vi "NI_SAT_TEST_20150519_EXP_V3_SINWAVE.vi"() -> ()   [LabVIEW 2013]
uses:
  <instrlib>/niFgen/niFgen.llb/niFgen Waveform Type.ctl
  <instrlib>/niFgen/niFgen.llb/niFgen Output Impedance.ctl
  <vilib>/Waveform/WDTOps.llb/WDT Append Waveforms DBL.vi
panel:
  out "appended array":dbl[](array[numeric])
  in  "amplitude":dbl=1.0 format="%#_3p"
  in  "frequency":dbl=1000000.0 format="%#_12p"
  in  "waveform":T1=5 caption="Waveform" items=["Sine", "Square", "Triangle", "Ramp Up", "Ramp Down", "DC", "Noise", "User"]
  out "Tabs 1 Through # Used":i32
  in  "Tab Control 3":T2(tab)
  out "Tab Control 2":T2(tab)
  out "Waveform Graph 1":waveform(dbl)(graph)
  out "Waveform Graph 2":waveform(dbl)(graph)
  out "Waveform Graph 3":waveform(dbl)(graph)
  out "Waveform Graph 4":waveform(dbl)(graph)
  out "Waveform Graph 5":waveform(dbl)(graph)
  out "Waveform Graph 6":waveform(dbl)(graph)
  out "Waveform Graph 7":waveform(dbl)(graph)
  out "Waveform Graph 8":waveform(dbl)(graph)
  out "Waveform Graph 9":waveform(dbl)(graph)
  out "Waveform Graph 10":waveform(dbl)(graph)
  out "Waveform Graph 11":waveform(dbl)(graph)
  out "Waveform Graph 12":waveform(dbl)(graph)
  out "Waveform Graph 13":waveform(dbl)(graph)
  out "Waveform Graph 14":waveform(dbl)(graph)
  out "Waveform Graph 15":waveform(dbl)(graph)
  out "Waveform Graph 16":waveform(dbl)(graph)
  out "Waveform Graph 17":waveform(dbl)(graph)
  out "Waveform Graph 18":waveform(dbl)(graph)
  out "Waveform Graph 19":waveform(dbl)(graph)
  out "Waveform Graph 20":waveform(dbl)(graph)
  out "Diff in Methods before call DMM vi and before read Wave Data (SEC)":dbl
  out "Total Elapsed Time (ms)":u32
  out "TotalElapsed Time (Sec)":dbl
  out "Waveform Graph":waveform(dbl)(graph)
  in  "Output Voltage Division":i32
  in  "Highest Output Voltage [Volts]":i32 min=-600 max=600 step=20
  in  "Rate":dbl=10.0 caption="Rate (Samples/Sec)" format="%.2f"
  in  "Waveform Points":i32=101 caption="Samples"
  in  "Function Generator Name":refnum<k15>="PXI1Slot2"
  # "Please Enter Output Voltage\nwith the desired sign. Be it positive\nor negative. Program will divide 200 and then negate, due to gain of 200 and inversion of input by amplifier"
  # "ENJOY PETER, still could use tweeking to make it run smoother and prevent more user error, but meh. Goodmorning"
  # "Output voltage comes from the VOLTAGE MONITOR (VM) from the amplifier with (1V VM/200V AMP)"
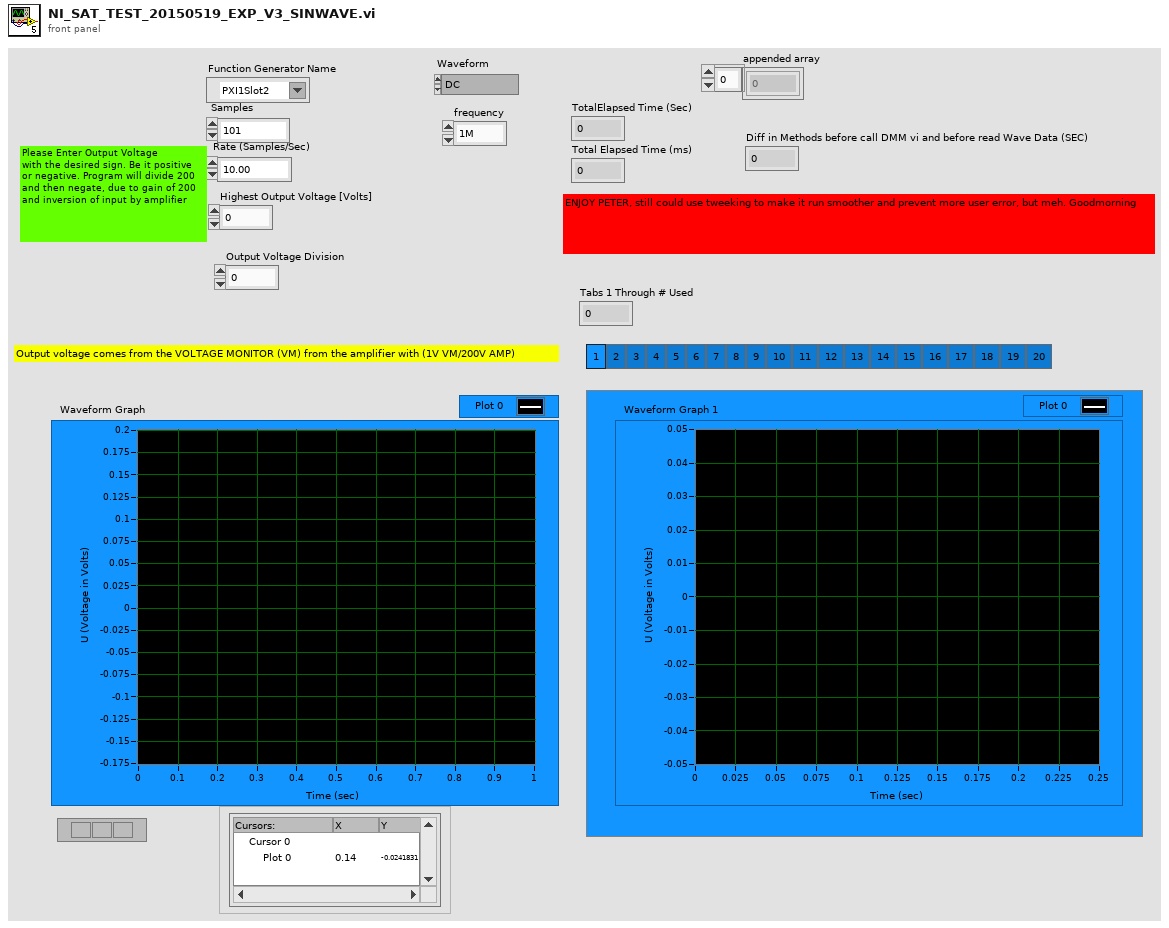
[diagram p1: front panel]
types:
  T1 = typedef "niFgen Waveform Type.ctl" = i32
  T2 = enum32{"1", "2", "3", "4", "5", "6", "7", "8", "9", "10", "11", "12", "13", "14", "15", "16", "17", "18", "19", "20"}
  T3 = enum16{"open", "replace", "create", "open or create", "replace or create", "replace or create with confirmation"}
  T4 = typedef "niFgen Output Impedance.ctl" = i32
  T5 = cluster{"channel name":string, "waveform":T1, "frequency":dbl, "y":dbl, "start phase":dbl, "dc offset":dbl, "duty cycle high":i32, "impedance":T4, "load impedance":dbl}
  T6 = cluster{"channel name":string, "waveform":T1, "frequency":dbl, "y":dbl, "start phase":dbl, "dc offset":dbl, "duty cycle high":i32, "impedance":T4, "load impedance":dbl}[]
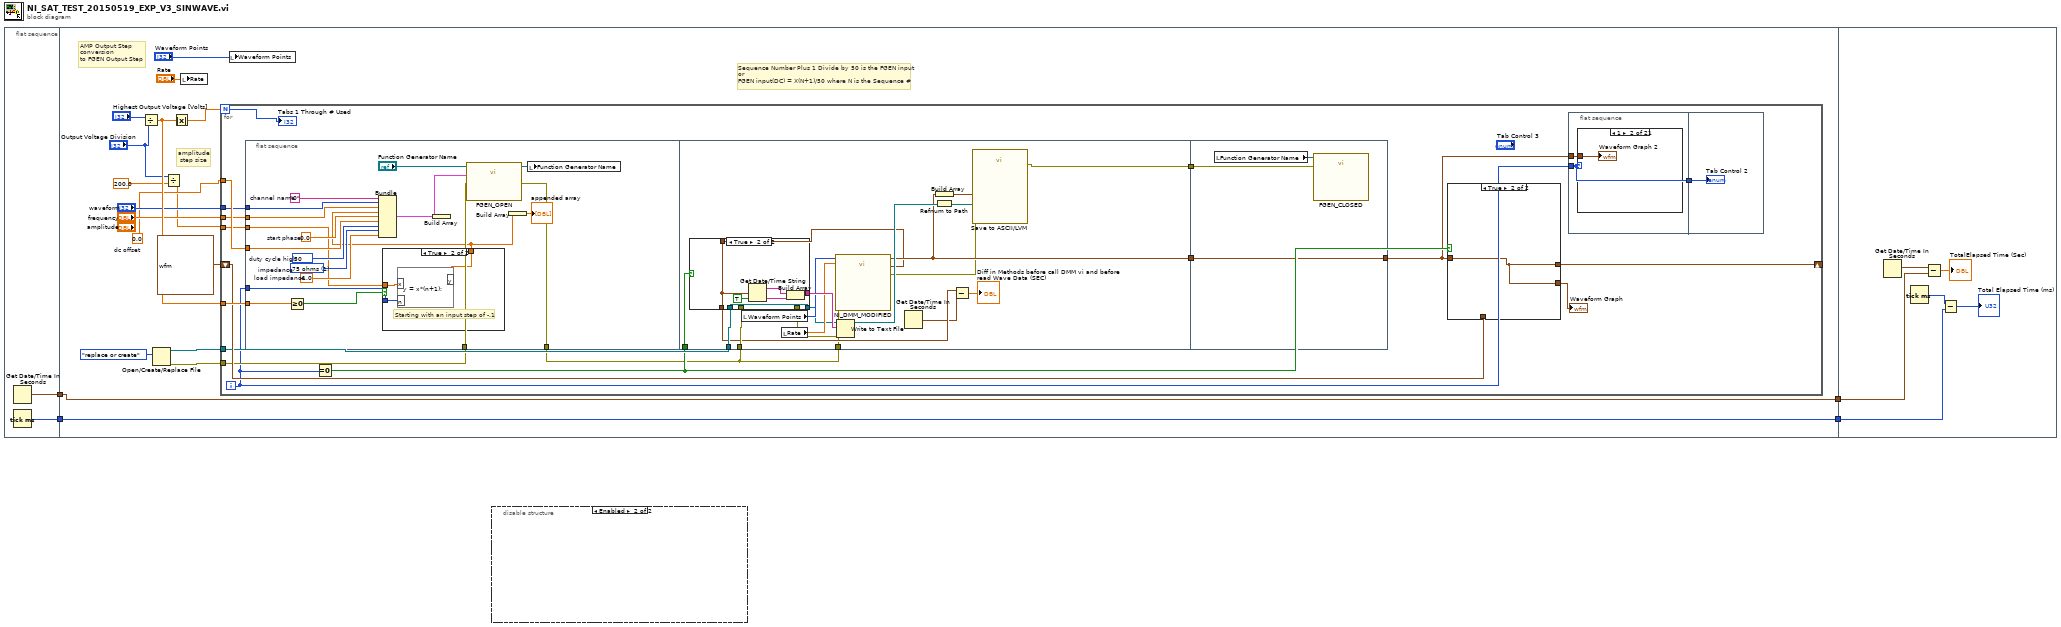
[diagram p0: block diagram]
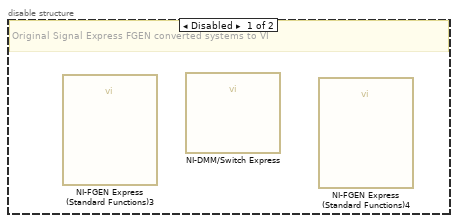
[diagram p2: hidden frame]
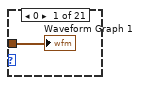
[diagram p3: hidden frame]
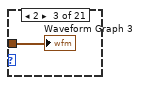
[diagram p4: hidden frame]
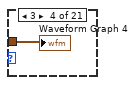
[diagram p5: hidden frame]
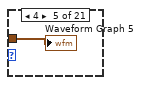
[diagram p6: hidden frame]
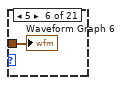
[diagram p7: hidden frame]
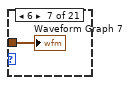
[diagram p8: hidden frame]
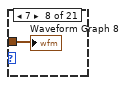
[diagram p9: hidden frame]
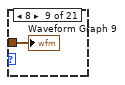
[diagram p10: hidden frame]
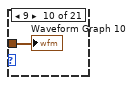
[diagram p11: hidden frame]
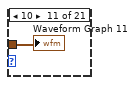
[diagram p12: hidden frame]
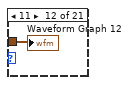
[diagram p13: hidden frame]
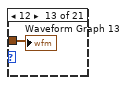
[diagram p14: hidden frame]
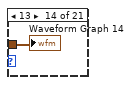
[diagram p15: hidden frame]
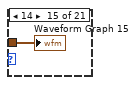
[diagram p16: hidden frame]
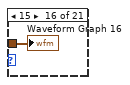
[diagram p17: hidden frame]
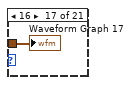
[diagram p18: hidden frame]
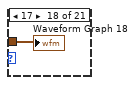
[diagram p19: hidden frame]
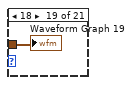
[diagram p20: hidden frame]
diagram:
  n1 = flat-sequence {
    tunnel: [w6] -> w4
    tunnel: [w5] -> w3
    tunnel: w4 -> [w15]
    tunnel: w3 -> [w14]
    tunnel: [w15] -> w2
    tunnel: [w14] -> w1
    tunnel: w2 -> [w136]
    tunnel: w1 -> [w135]
    frame #0 {
      n2 = Get Date/Time In Seconds() -> (seconds since 1Jan1904=w6:timestamp)
      n3 = Tick Count (ms)() -> (millisecond timer value=w5:u32)
    }
    frame #1 {
      w9 = 0.0  # dc offset
      # "AMP Output Step\nconversion\nto FGEN Output Step"
      # "amplitude\n step size"
      # "Sequence Number Plus 1 Divide by 50 is the FGEN input\nor\nFGEN input(DC) = X(N+1)/50 where N is the Sequence #"
      n4 = Divide(x="Highest Output Voltage [Volts]", y="Output Voltage Division") -> (x/y=w13:dbl)
      n5 = Open/Create/Replace File(operation (0:open)=T3."replace or create") -> (refnum out=w23:refnum<file>, error out=w22:errorcluster)  [unwired: 5 in, 1 out]
      n6 = Divide(x="Output Voltage Division", y=200.0) -> (x/y=w8:dbl)
      n7 = Absolute Value(x=w13) -> (abs(x)=w17:dbl)
      n8 = local write "Rate"("Rate") -> ()
      n9 = for {
        N: w17 -> [w29]
        tunnel: w23 -> [w37]
        tunnel: w22 -> [w34]
        tunnel: w13 -> [w40]
        shift-right: [w32] -> _
        shift-left: waveform(dbl) {"t0"=timestamp(0 s since 1904-01-01), "dt"=1.0, "Y"=[]} ("Waveform Data") -> [w39]
        tunnel: w9 -> [w27]
        tunnel: "waveform" -> [w26]
        tunnel: "frequency" -> [w25]
        tunnel: w8 -> [w24]
        i -> [w30]
        n10 = flat-sequence {
          tunnel: w30 -> [w82]
          tunnel: w40 -> [w79]
          tunnel: w34 -> [w77]
          tunnel: [w76] -> w33
          tunnel: w27 -> [w73]
          tunnel: w26 -> [w75]
          tunnel: w25 -> [w74]
          tunnel: w24 -> [w72]
          tunnel: [w109] -> w41
          tunnel: w36 -> [w106]
          tunnel: w37 -> [w105]
          tunnel: w33 -> [w103]
          tunnel: [w100] -> w35
          tunnel: w33 -> [w96]
          tunnel: w41 -> [w133]
          tunnel: [w133] -> w31
          tunnel: w35 -> [w132]
          frame #0 {
            w83 = -1.0  # load impedance
            w84 = T4 1 items=["50 ohms", "75 ohms", "1 mega ohm"]  # impedance
            w85 = 50  # duty cycle high
            w86 = 0.0  # start phase
            w71 = "0"  # channel name
            n11 = Greater Or Equal To 0?(x=w79) -> (x >= 0?=w78:bool)
            n12 = case shown="True" w78 {
              tunnel: w82 -> [w91 w94]
              tunnel: [w90 w93] -> w70
              tunnel: w72 -> [w89 w92]
              frame False {
                # "Starting with an input step of .1"
                # "Negative Output"
                n13 = formula code="y = -x*(n+1);"("x"=w89, "n"=w91) -> ("y"=w90:dbl)
              }
              frame True {
                # "Starting with an input step of -.1"
                n14 = formula code="y = x*(n+1);"("x"=w92, "n"=w94) -> ("y"=w93:dbl)
              }
            }
            n15 = Bundle("channel name"=w71, "waveform"=w75, "frequency"=w74, "y"=w70, "start phase"=w86, "dc offset"=w73, "duty cycle high"=w85, "impedance"=w84, "load impedance"=w83) -> (w81:T5)  [unwired: 1 in]
            n16 = Build Array(w81) -> (w80:T6)
            n17 = call "FGEN_OPEN.vi"("error in"=w77, "channel parameters"=w80, "resource name"="Function Generator Name") -> ("error out"=w76:errorcluster, "Instrument Handle Out"=w88:refnum<k15>)  [unwired: 7 in]
            n18 = Build Array(w70) -> (→"appended array":dbl[])
            n19 = local write "Function Generator Name"(w88) -> ()
          }
          frame #1 {
            n20 = local read "Waveform Points"() -> (w108:i32)
            n21 = local read "Rate"() -> (w107:dbl)
            n22 = call "NI_DMM_MODIFIED.vi"("Waveform Points"=w108, "Rate"=w107, "error in"=w96) -> ("Waveform Data"=w109:waveform(dbl), "current time"=w97:timestamp, "error out"=w101:errorcluster)  [unwired: 14 in]
            n23 = case shown="True" w106 {
              tunnel: [w120 w128] -> w113
              tunnel: w105 -> [w118 w127]
              tunnel: [w116 w127] -> w104
              tunnel: w103 -> [w117 w126]
              tunnel: [w115 w126] -> w102
              tunnel: [w114 w125] -> w99
              tunnel: w97 -> [w114 w125]
              frame False {
                n24 = Get Date/Time String(seconds (now)=w114, want seconds? (F)=TRUE) -> (date string=w123:string, time string=w122:string)  [unwired: 1 in]
                n25 = Set File Position(refnum=w118, from (0:start)=enum16{"start", "end", "current"}."end", error in=w117) -> (refnum out=w116:refnum<file>, error out=w115:errorcluster)  [unwired: 1 in]
                n26 = Build Array("" ("element"), w123, w122) -> (w120:string[])
              }
              frame True {
                n27 = Get Date/Time String(seconds (now)=w125, want seconds? (F)=TRUE) -> (date string=w130:string, time string=w129:string)  [unwired: 1 in]
                n28 = Build Array(w130, w129) -> (w128:string[])
              }
            }
            n29 = Write to Text File(file (use dialog)=w104, text=w113, error in=w102) -> (refnum out=w112:refnum<file>)  [unwired: 1 in, 2 out]
            n30 = Get Date/Time In Seconds() -> (seconds since 1Jan1904=w95:timestamp)
            n31 = Build Array(w109) -> (w110:waveform(dbl)[])
            n32 = Refnum to Path(1:w112) -> (0:w111:path)
            n33 = Subtract(x=w99, y=w95) -> (x-y=→"Diff in Methods before call DMM vi and before read Wave Data (SEC)":dbl)
            n34 = call "Save to ASCII/LVM"("signals in"=w110, "File Path"=w111, "error in"=w101) -> ("error out"=w100:errorcluster)  [unwired: 16 in]
          }
          frame #2 {
            n35 = local read "Function Generator Name"() -> (w134:refnum<k15>)
            n36 = call "FGEN_CLOSED.vi"("error in"=w132, "instrument handle"=w134) -> ()  [unwired: 9 in, 1 out]
          }
        }
        n37 = Equal To 0?(x=w30) -> (x = 0?=w36:bool)
        n38 = case shown="True" w36 {
          tunnel: w31 -> [w65 w68]
          tunnel: [w66 w68] -> w32
          tunnel: w39 -> [w67 _]
          tunnel: [w66 w68] -> w38
          frame False {
            n39 = call-poly <vilib>:"Append Waveforms.vi"("waveform B"=w65, "waveform A"=w67) -> ("waveform out"=w66:waveform(dbl))  [unwired: 8 in, 1 out]
          }
          frame True {
          }
        }
        "Waveform Graph" <- w38
        n40 = flat-sequence {
          tunnel: w31 -> [w43]
          tunnel: w30 -> [w42]
          tunnel: [w42] -> w28
          tunnel: w28 -> [w64]
          frame #0 {
            n41 = case shown="1" w42 {
              tunnel: w43 -> [w44 w45 w46 w47 w48 w49 w50 w51 w52 w53 w54 w55 w56 w57 w58 w59 w60 w61 w62 w63 _]
              frame 0 {
                "Waveform Graph 1" <- w44
              }
              frame 1 {
                "Waveform Graph 2" <- w45
              }
              frame 2 {
                "Waveform Graph 3" <- w46
              }
              frame 3 {
                "Waveform Graph 4" <- w47
              }
              frame 4 {
                "Waveform Graph 5" <- w48
              }
              frame 5 {
                "Waveform Graph 6" <- w49
              }
              frame 6 {
                "Waveform Graph 7" <- w50
              }
              frame 7 {
                "Waveform Graph 8" <- w51
              }
              frame 8 {
                "Waveform Graph 9" <- w52
              }
              frame 9 {
                "Waveform Graph 10" <- w53
              }
              frame 10 {
                "Waveform Graph 11" <- w54
              }
              frame 11 {
                "Waveform Graph 12" <- w55
              }
              frame 12 {
                "Waveform Graph 13" <- w56
              }
              frame 13 {
                "Waveform Graph 14" <- w57
              }
              frame 14 {
                "Waveform Graph 15" <- w58
              }
              frame 15 {
                "Waveform Graph 16" <- w59
              }
              frame 16 {
                "Waveform Graph 17" <- w60
              }
              frame 17 {
                "Waveform Graph 18" <- w61
              }
              frame 18 {
                "Waveform Graph 19" <- w62
              }
              frame 19 {
                "Waveform Graph 20" <- w63
              }
              frame 20, Default {
              }
            }
          }
          frame #1 {
            "Tab Control 2" <- w64
          }
        }
        "Tabs 1 Through # Used" <- w29
      }
      n42 = local write "Waveform Points"("Waveform Points") -> ()
    }
    frame #2 {
      n43 = Get Date/Time In Seconds() -> (seconds since 1Jan1904=w137:timestamp)
      n44 = Tick Count (ms)() -> (millisecond timer value=w139:u32)
      n45 = Subtract(x=w137, y=w136) -> (x-y=→"TotalElapsed Time (Sec)":dbl)
      n46 = Subtract(x=w139, y=w135) -> (x-y=→"Total Elapsed Time (ms)":u32)
    }
  }
  n47 = disable-structure shown="Enabled" {
    frame Disabled {
      # "Original Signal Express FGEN converted systems to VI"
      n48 = call "NI-FGEN Express (Standard Functions)3"() -> ()  [unwired: 11 in, 1 out]
      n49 = call "NI-DMM/Switch Express"() -> ()  [unwired: 17 in, 3 out]
      n50 = call "NI-FGEN Express (Standard Functions)4"() -> ()  [unwired: 11 in, 1 out]
    }
    frame Enabled {
    }
  }
